vi "RSZVB Get Calibration Data Parameters More Calibrations.vi"(0 "VISA session":refnum<visa-resource-name>, 5 "Channel (1)":i32=1, 7 "Calibration (1)":i32=1, 11 "error in (no error)":errorcluster {"code" format="%.0x"}) -> (3 "Sweep Type":i32, 4 "dup VISA session":refnum<visa-resource-name>, 6 "Frequency Start":dbl format="%^.3e", 8 "Frequency Stop":dbl format="%^.3e", 10 "Number Of Points":i32, 14 "Internal Signal Source Power":dbl format="%^.3e", 15 "error out":errorcluster {"code" format="%.0x"})   [LabVIEW 2011]
doc: "This VI queries the parameters of the channel's calibration\n\nRemote-control command(s):\n[SENSe<Ch>:]CORRection:DATA:PARameter<Cal>?"
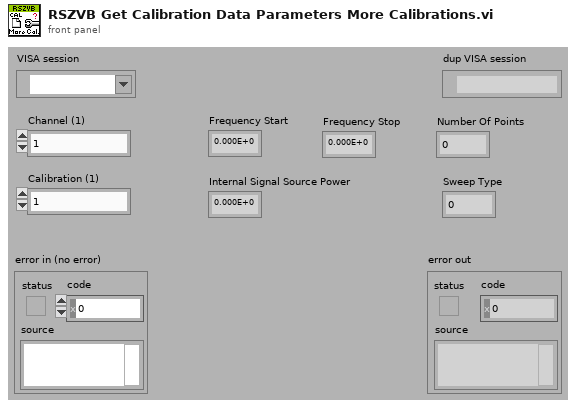
[diagram p1: front panel]
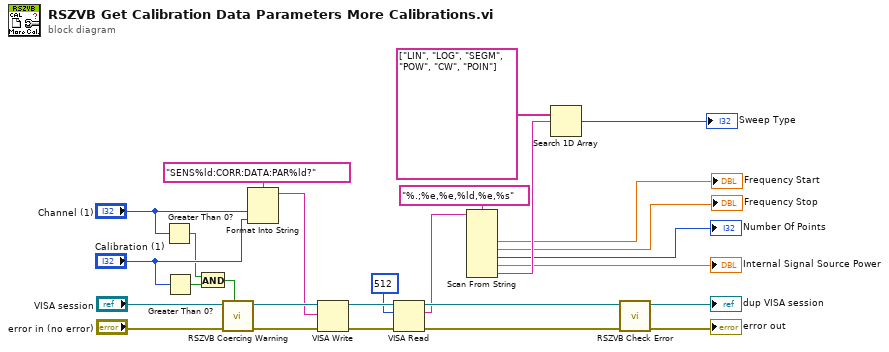
[diagram p0: block diagram]
diagram:
  n1 = Greater Than 0?(x="Channel (1)") -> (x > 0?=w2:bool)
  n2 = Greater Than 0?(x="Calibration (1)") -> (x > 0?=w3:bool)
  n3 = And(x=w2, y=w3) -> (x .and. y?=w1:bool)
  n4 = call "RSZVB Coercing Warning.vi"("In Range?"=w1, "error in (no error)"="error in (no error)", "VISA session"="VISA session") -> ("error out"=w26:errorcluster, "dup VISA session"=w27:refnum<visa-resource-name>)  [unwired: 7 in]
  n5 = Format Into String(format string="SENS%ld:CORR:DATA:PAR%ld?", "Channel (1)", "Calibration (1)") -> (resulting string=w20:string)  [unwired: 2 in, 1 out]
  n6 = VISA Write(VISA resource name=w27, write buffer=w20, error in (no error)=w26) -> (VISA resource name out=w25:refnum<visa-resource-name>, error out=w24:errorcluster)  [unwired: 1 out]
  n7 = VISA Read(VISA resource name=w25, byte count=u32 512 ("byte count (0)"), error in (no error)=w24) -> (VISA resource name out=w23:refnum<visa-resource-name>, read buffer=w18:string, error out=w22:errorcluster)  [unwired: 1 out]
  n8 = Scan From String(format string="%.;%e,%e,%ld,%e,%s", input string=w18) -> (output 1=→"Frequency Start":dbl, output 2=→"Frequency Stop":dbl, output 3=→"Number Of Points":i32, output 4=→"Internal Signal Source Power":dbl, output 5=w15:string)  [unwired: 7 in, 3 out]
  n9 = Search 1D Array(1D array=string[] ["LIN", "LOG", "SEGM", "POW", "CW", "POIN"], element=w15) -> (index of element=→"Sweep Type":i32)  [unwired: 1 in]
  n10 = call "RSZVB Check Error.vi"("error in (no error)"=w22, "VISA session"=w23) -> ("error out"=→"error out":errorcluster, "dup VISA session"=→"dup VISA session":refnum<visa-resource-name>)  [unwired: 8 in]
